vi "Write_read_uart esp-32 (SubVI).vi"(4 "error in (no error)":errorcluster, 5 "write buffer":string="c/gpio/out/high/pin:19\n", 6 "milliseconds to wait":u32=50, 7 "VISA Refnum in":refnum<visa-resource-name>="COM7") -> (0 "error out 4":errorcluster, 1 "read buffer":string, 2 "read bite":u32, 3 "VISA resource name out":refnum<visa-resource-name>)   [LabVIEW 2018]
panel:
  out "error out 3":errorcluster
  out "write bite":u32
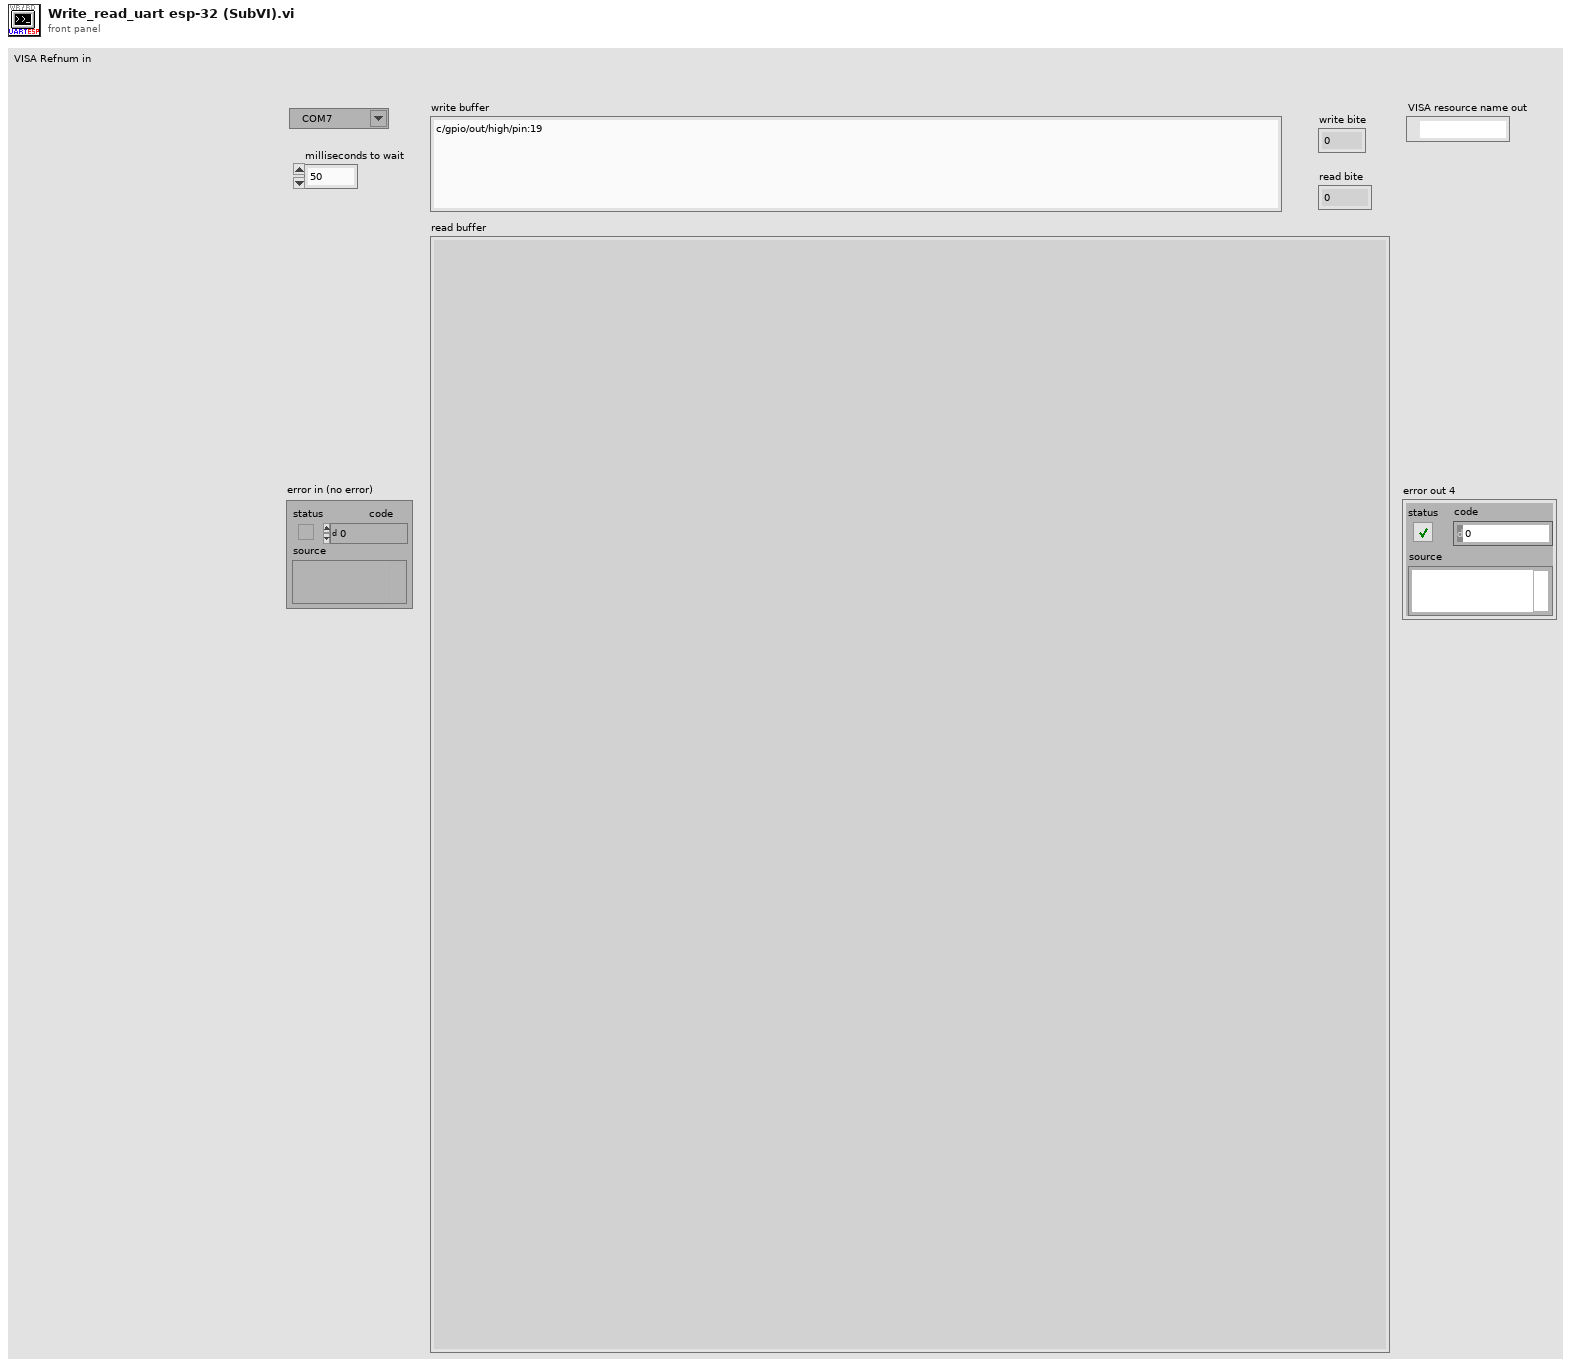
[diagram p1: front panel]
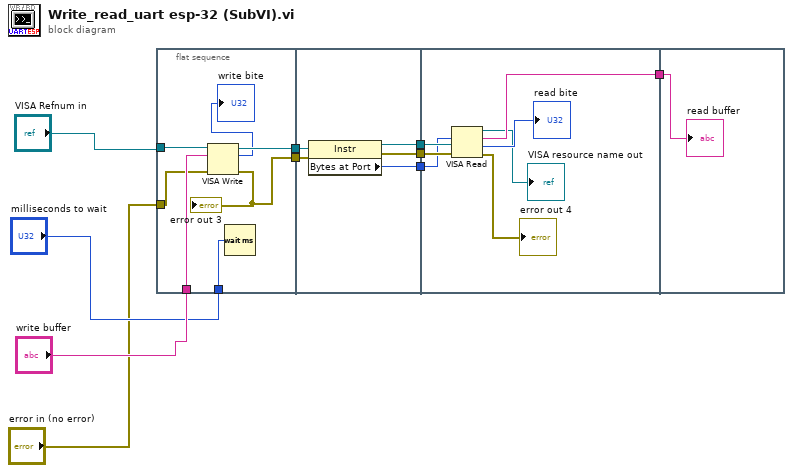
[diagram p0: block diagram]
diagram:
  n1 = flat-sequence {
    tunnel: [w17] -> w10
    tunnel: [w16] -> w9
    tunnel: "write buffer" -> [w14]
    tunnel: "milliseconds to wait" -> [w13]
    tunnel: "VISA Refnum in" -> [w12]
    tunnel: "error in (no error)" -> [w11]
    tunnel: w10 -> [w21]
    tunnel: w9 -> [w22]
    tunnel: [w20] -> w8
    tunnel: [w19] -> w7
    tunnel: [w18] -> w6
    tunnel: w8 -> [w27]
    tunnel: w7 -> [w28]
    tunnel: w6 -> [w24]
    tunnel: [w25] -> w5
    tunnel: w5 -> [w30]
    frame #0 {
      n2 = VISA Write(VISA resource name=w12, write buffer=w14, error in (no error)=w11) -> (VISA resource name out=w16:refnum<visa-resource-name>, return count=→"write bite":u32, error out=w17:errorcluster)
      "error out 3" <- w17
      n3 = Wait (ms)(milliseconds to wait=w13) -> ()  [unwired: 1 out]
    }
    frame #1 {
      n4 = property class="Instr"(reference=w22, error in=w21) -> (reference out=w20:refnum<visa-resource-name>, error out=w19:errorcluster, "Bytes at Port"=w18:u32)
    }
    frame #2 {
      n5 = VISA Read(VISA resource name=w27, byte count=w24, error in (no error)=w28) -> (VISA resource name out=→"VISA resource name out":refnum<visa-resource-name>, read buffer=w25:string, return count=→"read bite":u32, error out=→"error out 4":errorcluster)
    }
    frame #3 {
      "read buffer" <- w30
    }
  }
